vi "test list.vi"() -> ()   [LabVIEW 2014]
uses:
  user.lib/_NEVSTOP/Communicable State Machine(CSM)/_Support/Priority Queue/Priority Queue.lvclass/Priority Queue.ctl
  user.lib/_NEVSTOP/Communicable State Machine(CSM)/Utility/uuid.vi
  user.lib/_NEVSTOP/Communicable State Machine(CSM)/_Support/Process/CSMP-Async Call.vi
  user.lib/_NEVSTOP/Communicable State Machine(CSM)/Utility/Trim Both Whitespace.vi
  user.lib/_NEVSTOP/Communicable State Machine(CSM)/_Support/CSMQ/_CSMObj-Message Check.vi
  user.lib/_NEVSTOP/Communicable State Machine(CSM)/_Support/CSMQ/_CSMObj-Enqueue Cross-Module Message.vi
  user.lib/_NEVSTOP/Communicable State Machine(CSM)/_Support/CSMQ/_CSMOFGV Get.vi
  user.lib/_NEVSTOP/Communicable State Machine(CSM)/_Support/Priority Queue/Enqueue Element.vi
  user.lib/_NEVSTOP/Communicable State Machine(CSM)/Utility/Build Error Cluster.vi
  user.lib/_NEVSTOP/Communicable State Machine(CSM)/_Support/CSMQ/_CSMOFGV.vi
  user.lib/_NEVSTOP/Communicable State Machine(CSM)/Communicable State Machine.lvlib
panel:
  out "Module Names 4":string[](array[string])
  out "Module Names 3":string[](array[string])
  out "Module Names 2":string[](array[string])
  out "Module Names":string[](array[string])
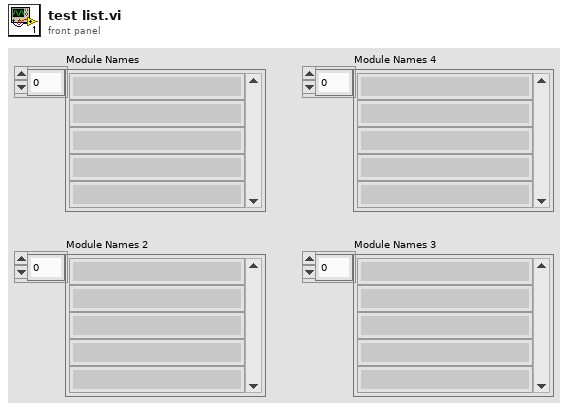
[diagram p1: front panel]
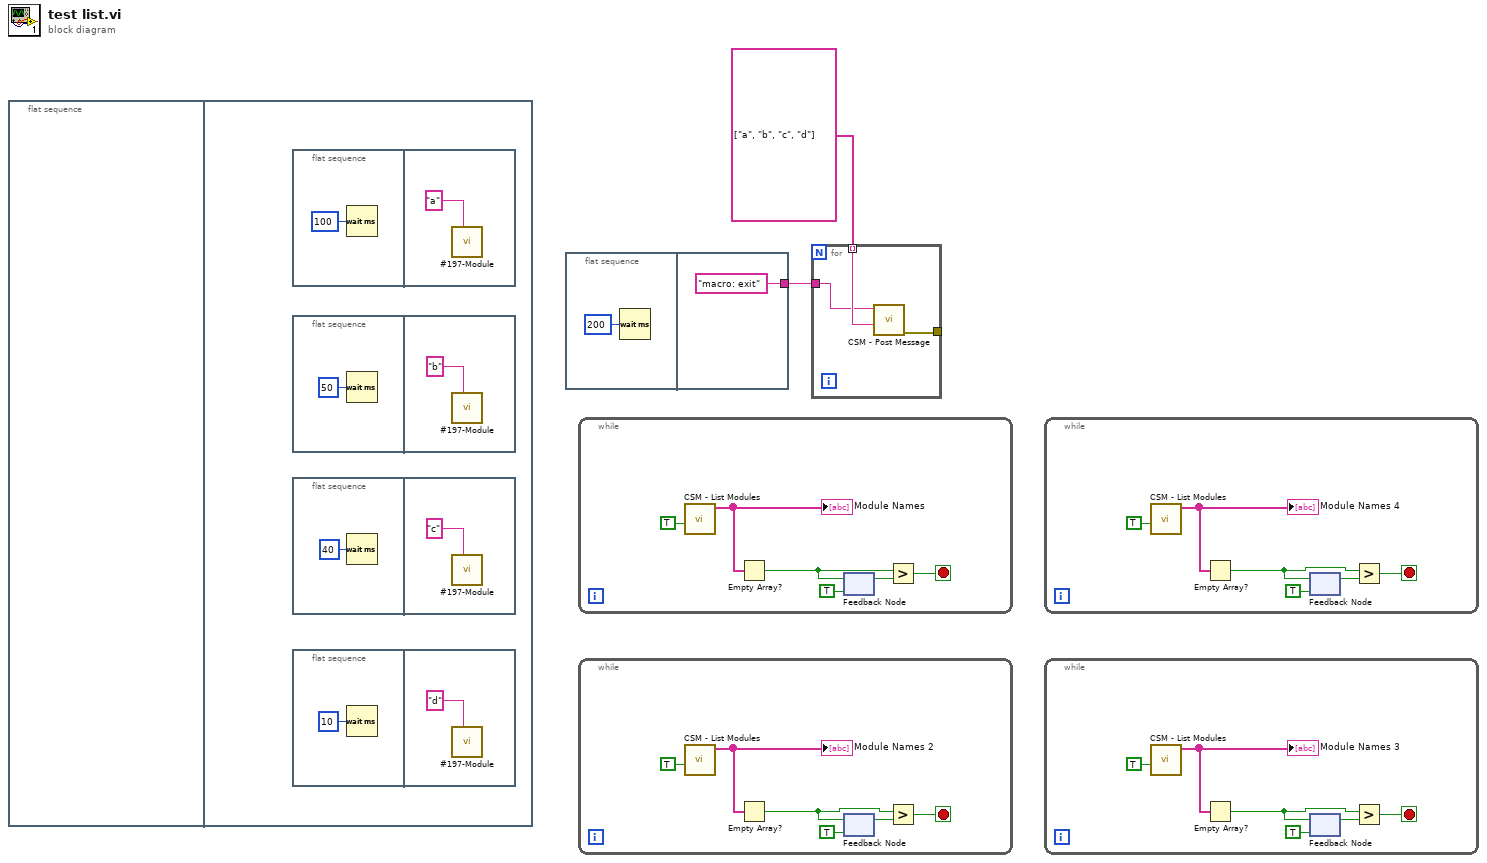
[diagram p0: block diagram]
diagram:
  n1 = flat-sequence {
    frame #0 {
    }
    frame #1 {
      n2 = flat-sequence {
        frame #0 {
          n3 = Wait (ms)(milliseconds to wait=u32 100) -> ()  [unwired: 1 out]
        }
        frame #1 {
          n4 = call "#197-Module.vi"("Name(\"\" to use uuid)"="a" ("Name(\"\" to use uuid)")) -> ()  [unwired: 11 in]
        }
      }
      n5 = flat-sequence {
        frame #0 {
          n6 = Wait (ms)(milliseconds to wait=u32 50) -> ()  [unwired: 1 out]
        }
        frame #1 {
          n7 = call "#197-Module.vi"("Name(\"\" to use uuid)"="b" ("Name(\"\" to use uuid)")) -> ()  [unwired: 11 in]
        }
      }
      n8 = flat-sequence {
        frame #0 {
          n9 = Wait (ms)(milliseconds to wait=u32 40) -> ()  [unwired: 1 out]
        }
        frame #1 {
          n10 = call "#197-Module.vi"("Name(\"\" to use uuid)"="c" ("Name(\"\" to use uuid)")) -> ()  [unwired: 11 in]
        }
      }
      n11 = flat-sequence {
        frame #0 {
          n12 = Wait (ms)(milliseconds to wait=u32 10) -> ()  [unwired: 1 out]
        }
        frame #1 {
          n13 = call "#197-Module.vi"("Name(\"\" to use uuid)"="d" ("Name(\"\" to use uuid)")) -> ()  [unwired: 11 in]
        }
      }
    }
  }
  n14 = flat-sequence {
    tunnel: ["macro: exit" ("State")] -> w1
    frame #0 {
      n15 = Wait (ms)(milliseconds to wait=u32 200) -> ()  [unwired: 1 out]
    }
    frame #1 {
    }
  }
  n16 = while {
    stop <- w14 stop-if-true
    n17 = call "CSM - List Modules.vi"("All?"=TRUE) -> ("Module Names"=w17:string[])  [unwired: 9 in, 1 out]
    "Module Names" <- w17
    n18 = Empty Array?(array=w17) -> (empty?=w13:bool)
    n19 = feedback-in #1(w13) -> ()
    n20 = feedback #1(TRUE ("empty?")) -> (w16:bool)
    n21 = Greater?(x=w13, y=w16) -> (0:w14:bool)
  }
  n22 = while {
    stop <- w20 stop-if-true
    n23 = call "CSM - List Modules.vi"("All?"=TRUE) -> ("Module Names"=w23:string[])  [unwired: 9 in, 1 out]
    "Module Names 2" <- w23
    n24 = Empty Array?(array=w23) -> (empty?=w19:bool)
    n25 = feedback-in #2(w19) -> ()
    n26 = feedback #2(TRUE ("empty?")) -> (w22:bool)
    n27 = Greater?(x=w19, y=w22) -> (0:w20:bool)
  }
  n28 = for {
    tunnel: [w27] -> _
    tunnel: string[] ["a", "b", "c", "d"] ("Module Names (in)") -> [w26] mode=indexing
    tunnel: w1 -> [w25]
    n29 = call "CSM - Post Message.vi"("Target Module"=w26, "State"=w25) -> ("error out"=w27:errorcluster)  [unwired: 9 in]
  }
  n30 = while {
    stop <- w29 stop-if-true
    n31 = call "CSM - List Modules.vi"("All?"=TRUE) -> ("Module Names"=w32:string[])  [unwired: 9 in, 1 out]
    "Module Names 4" <- w32
    n32 = Empty Array?(array=w32) -> (empty?=w28:bool)
    n33 = feedback-in #3(w28) -> ()
    n34 = feedback #3(TRUE ("empty?")) -> (w31:bool)
    n35 = Greater?(x=w28, y=w31) -> (0:w29:bool)
  }
  n36 = while {
    stop <- w35 stop-if-true
    n37 = call "CSM - List Modules.vi"("All?"=TRUE) -> ("Module Names"=w38:string[])  [unwired: 9 in, 1 out]
    "Module Names 3" <- w38
    n38 = Empty Array?(array=w38) -> (empty?=w34:bool)
    n39 = feedback-in #4(w34) -> ()
    n40 = feedback #4(TRUE ("empty?")) -> (w37:bool)
    n41 = Greater?(x=w34, y=w37) -> (0:w35:bool)
  }
